vi "ICG_YY.vi"() -> ()   [LabVIEW 2020]
uses:
  <vilib>/Utility/file.llb/Read Delimited Spreadsheet (DBL).vi
  <vilib>/Analysis/NI_AALPro.lvlib
panel:
  out "size(s)":i32
  out "SV 4":dbl
  out "SV 3":dbl
  out "SV 2":dbl
  out "SV":dbl
  out "SV":dbl
  out "Tlve 5":dbl
  out "interval7 2":dbl[](graph)
  out "location 5":dbl[](array[numeric])
  out "interval 7":dbl[](array[numeric])
  out "amplitude 5":dbl[](array[numeric])
  out "Amplitudes 5":dbl[](array[numeric])
  out "2nd Derivatives 5":dbl[](array[numeric])
  out "Locations 5":dbl[](array[numeric])
  out "max  4":dbl
  out "deltaZe(t)4 2":dbl[](graph)
  out "ICG array 5":dbl[](array[numeric])
  in  "file path (dialog if empty) 5":path
  out "Tlve 4":dbl
  out "interval7":dbl[](graph)
  out "location 4":dbl[](array[numeric])
  out "interval 6":dbl[](array[numeric])
  out "amplitude 4":dbl[](array[numeric])
  out "Amplitudes 4":dbl[](array[numeric])
  out "2nd Derivatives 4":dbl[](array[numeric])
  out "Locations 4":dbl[](array[numeric])
  out "max  3":dbl
  out "deltaZe(t)4":dbl[](graph)
  out "ICG array 4":dbl[](array[numeric])
  in  "file path (dialog if empty) 4":path
  out "Tlve 3":dbl
  out "interval 5":dbl[](graph)
  out "location 3":dbl[](array[numeric])
  out "interval 4":dbl[](array[numeric])
  out "amplitude 3":dbl[](array[numeric])
  out "Amplitudes 3":dbl[](array[numeric])
  out "2nd Derivatives 3":dbl[](array[numeric])
  out "Locations 3":dbl[](array[numeric])
  out "max  2":dbl
  out "deltaZe(t) 3":dbl[](graph)
  out "ICG array 3":dbl[](array[numeric])
  in  "file path (dialog if empty) 3":path
  out "Tlve 2":dbl
  out "interval 3":dbl[](graph)
  out "location 2":dbl[](array[numeric])
  out "interval 2":dbl[](array[numeric])
  out "amplitude 2":dbl[](array[numeric])
  out "Amplitudes 2":dbl[](array[numeric])
  out "2nd Derivatives 2":dbl[](array[numeric])
  out "Locations 2":dbl[](array[numeric])
  out "max  2":dbl
  out "deltaZe(t) 2":dbl[](graph)
  out "ICG":dbl[](array[numeric])
  in  "file path (dialog if empty) 2":path
  out "Tlve":dbl
  out "interval":dbl[](graph)
  out "location":dbl[](array[numeric])
  out "interval":dbl[](array[numeric])
  out "amplitude":dbl[](array[numeric])
  out "Amplitudes":dbl[](array[numeric])
  out "2nd Derivatives":dbl[](array[numeric])
  out "Locations":dbl[](array[numeric])
  out "max":dbl
  out "deltaZe(t)":dbl[](graph)
  out "ICG":dbl[](array[numeric])
  in  "file path (dialog if empty)":path
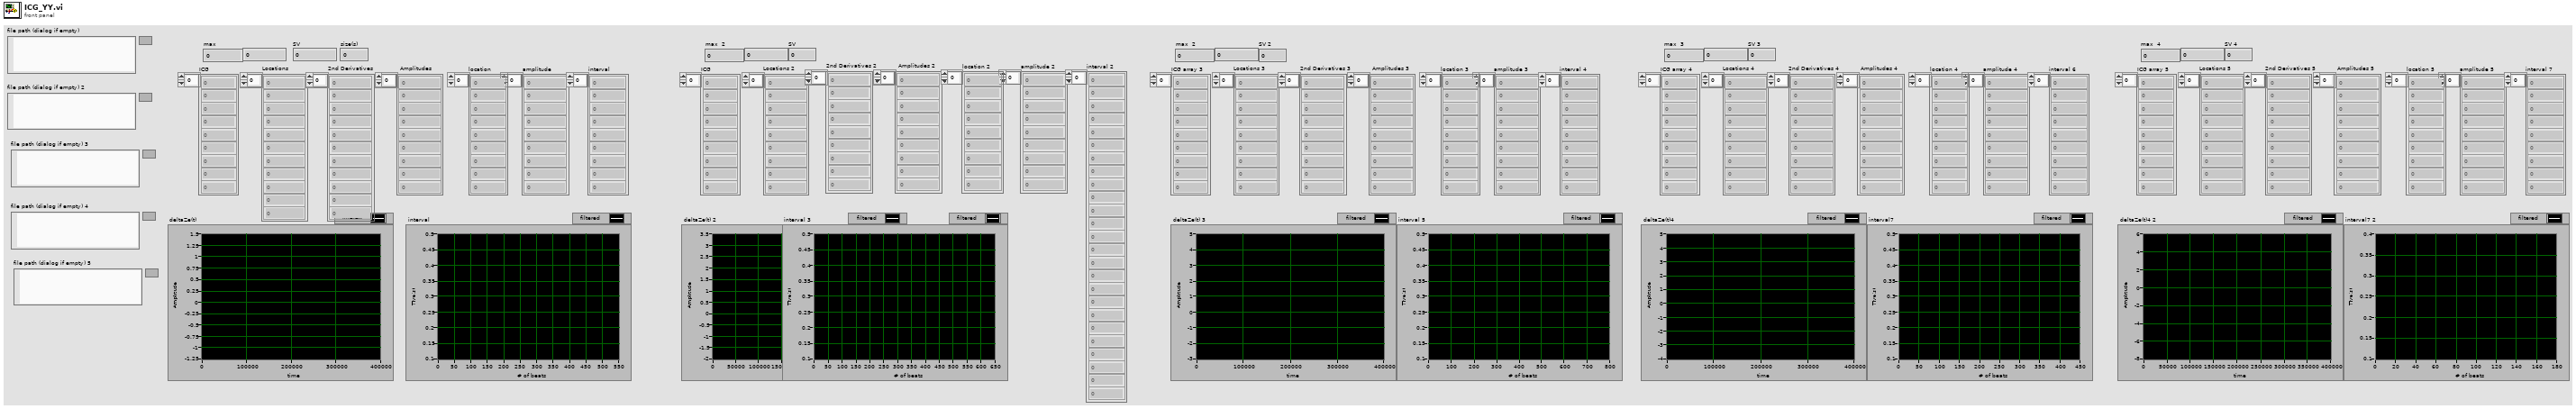
[diagram p1: front panel]
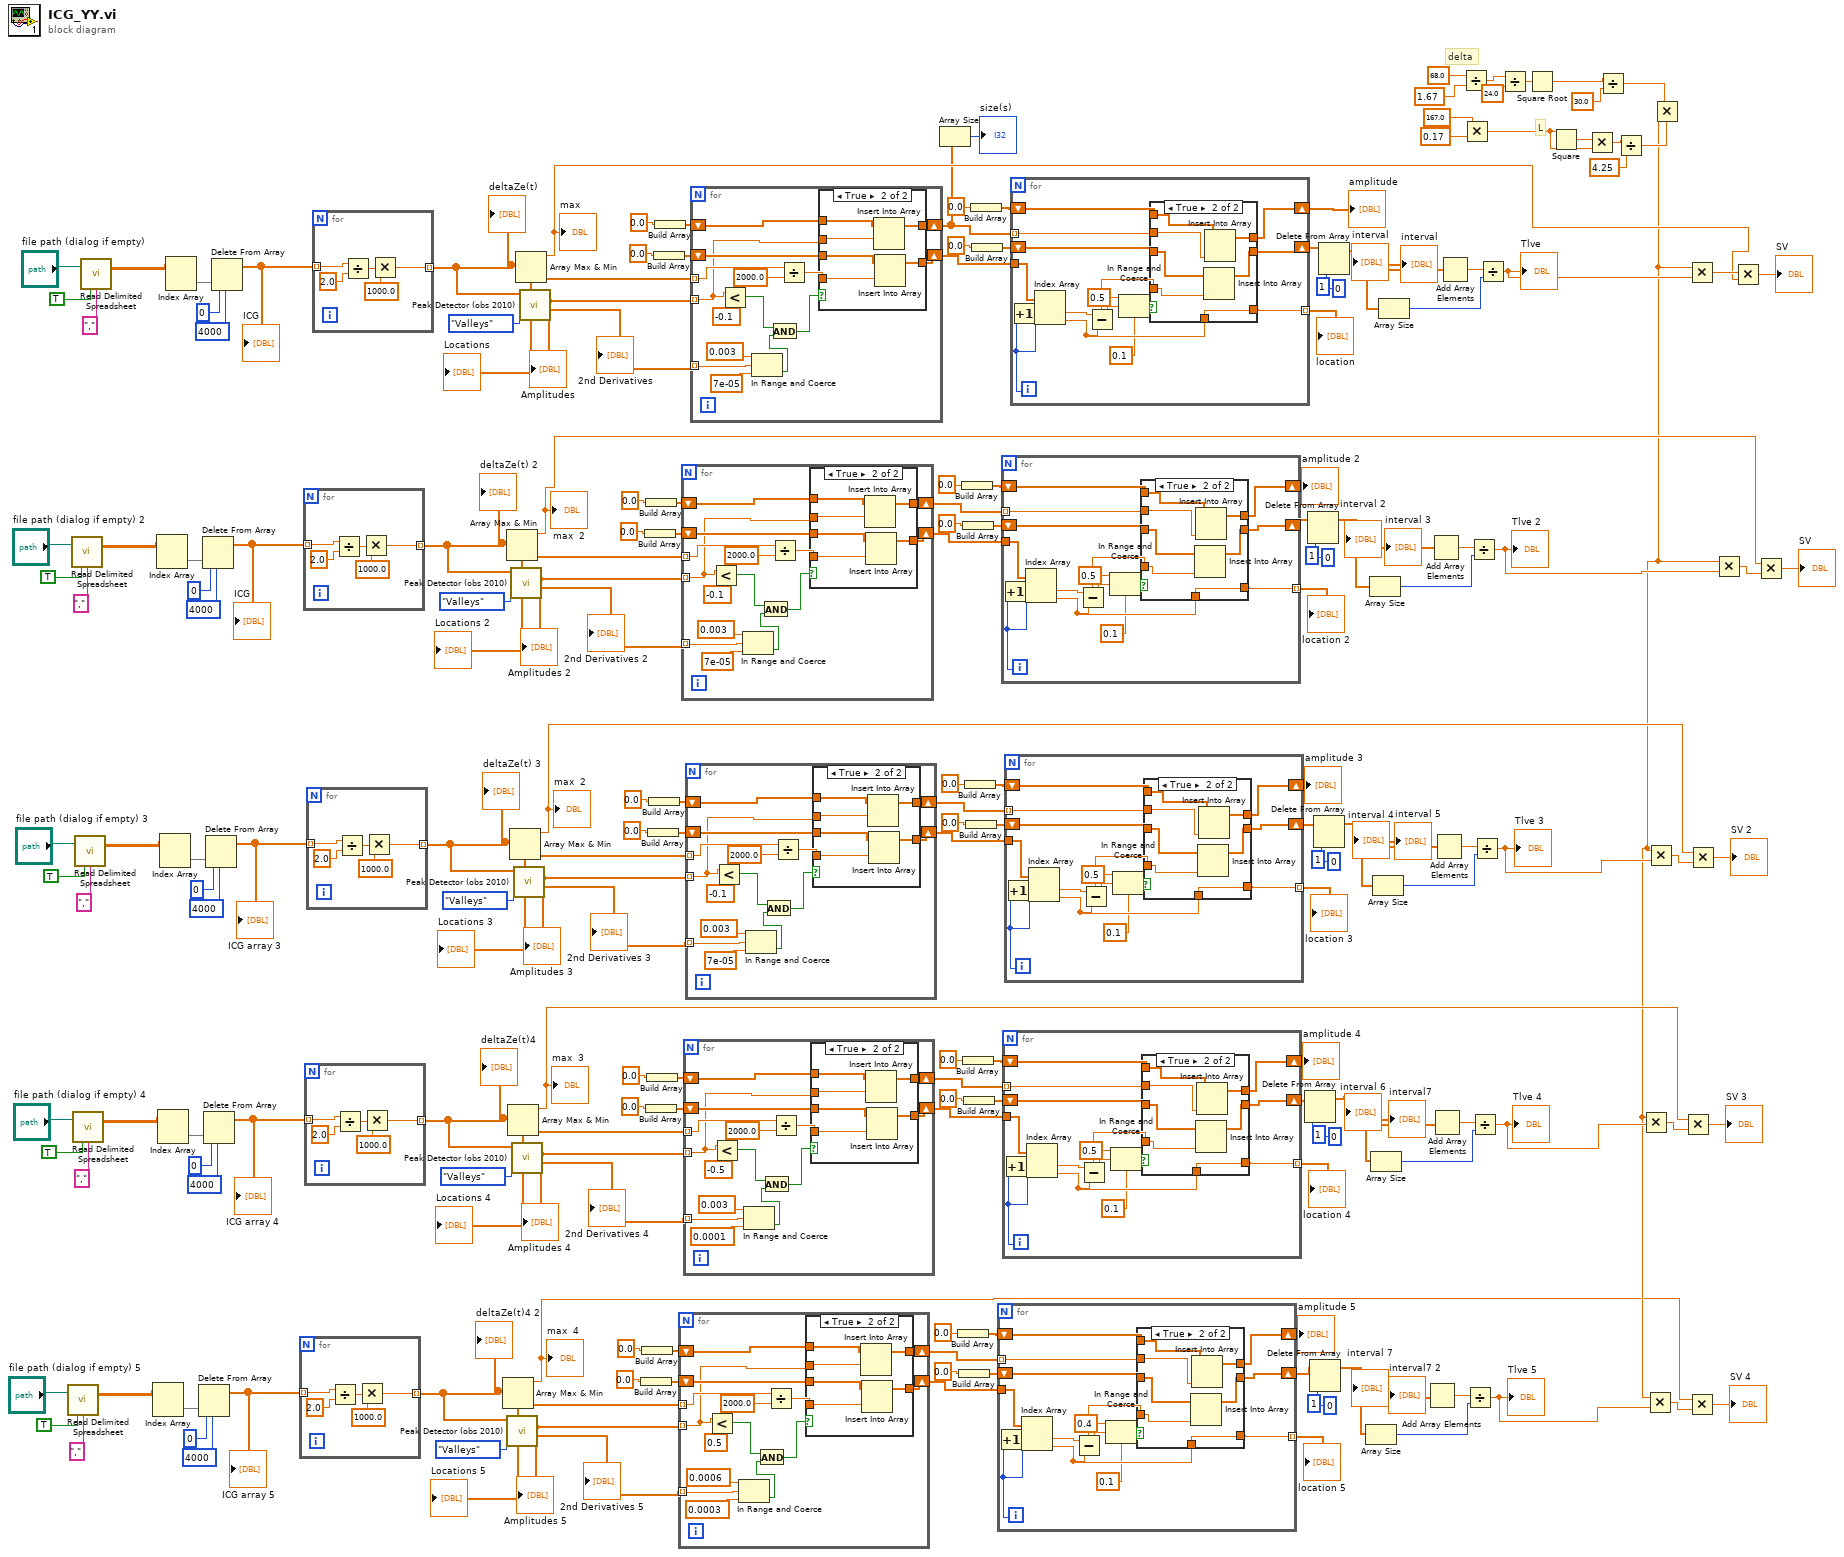
[diagram p0: block diagram]
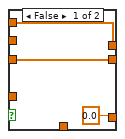
[diagram p2: hidden frame]
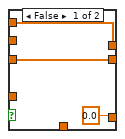
[diagram p4: hidden frame]
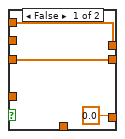
[diagram p6: hidden frame]
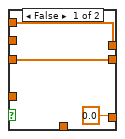
[diagram p8: hidden frame]
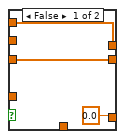
[diagram p10: hidden frame]
diagram:
  (unwired) 1 ("length")
  (unwired) 1 ("length")
  (unwired) 1 ("length")
  (unwired) 1 ("length")
  (unwired) 1 ("length")
  # "L"
  # "delta"
  n1 = call-poly <vilib>:"Read Delimited Spreadsheet.vi"("file path (dialog if empty)"="file path (dialog if empty) 5", "transpose? (F)"=TRUE, "delimiter (\\t)"="," ("delimiter (\\t)")) -> ("all rows"=w77:dbl[][])  [unwired: 7 in, 5 out]
  n2 = call-poly <vilib>:"Read Delimited Spreadsheet.vi"("file path (dialog if empty)"="file path (dialog if empty) 2", "transpose? (F)"=TRUE, "delimiter (\\t)"="," ("delimiter (\\t)")) -> ("all rows"=w158:dbl[][])  [unwired: 7 in, 5 out]
  n3 = call-poly <vilib>:"Read Delimited Spreadsheet.vi"("file path (dialog if empty)"="file path (dialog if empty) 4", "transpose? (F)"=TRUE, "delimiter (\\t)"="," ("delimiter (\\t)")) -> ("all rows"=w104:dbl[][])  [unwired: 7 in, 5 out]
  n4 = call-poly <vilib>:"Read Delimited Spreadsheet.vi"("file path (dialog if empty)"="file path (dialog if empty) 3", "transpose? (F)"=TRUE, "delimiter (\\t)"="," ("delimiter (\\t)")) -> ("all rows"=w131:dbl[][])  [unwired: 7 in, 5 out]
  n5 = call-poly <vilib>:"Read Delimited Spreadsheet.vi"("file path (dialog if empty)"="file path (dialog if empty)", "transpose? (F)"=TRUE, "delimiter (\\t)"="," ("delimiter (\\t)")) -> ("all rows"=w184:dbl[][])  [unwired: 7 in, 5 out]
  n6 = Index Array(array=w77) -> (element=w76:dbl[])  [unwired: 2 in]
  n7 = Index Array(array=w158) -> (element=w157:dbl[])  [unwired: 2 in]
  n8 = Index Array(array=w104) -> (element=w103:dbl[])  [unwired: 2 in]
  n9 = Index Array(array=w131) -> (element=w130:dbl[])  [unwired: 2 in]
  n10 = Index Array(array=w184) -> (element=w183:dbl[])  [unwired: 2 in]
  n11 = Delete From Array(array=w76, length=4000, index=0) -> (array with subset deleted=w73:dbl[])  [unwired: 1 out]
  "ICG array 5" <- w73
  n12 = Delete From Array(array=w157, length=4000, index=0) -> (array with subset deleted=w154:dbl[])  [unwired: 1 out]
  "ICG" <- w154
  n13 = Delete From Array(array=w103, length=4000, index=0) -> (array with subset deleted=w100:dbl[])  [unwired: 1 out]
  "ICG array 4" <- w100
  n14 = Delete From Array(array=w130, length=4000, index=0) -> (array with subset deleted=w127:dbl[])  [unwired: 1 out]
  "ICG array 3" <- w127
  n15 = Delete From Array(array=w183, length=4000, index=0) -> (array with subset deleted=w180:dbl[])  [unwired: 1 out]
  "ICG" <- w180
  n16 = for {
    tunnel: w73 -> [w192] mode=indexing
    tunnel: [w188] -> w69 mode=indexing
    n17 = Divide(x=w192, y=2.0) -> (x/y=w190:dbl)
    n18 = Multiply(x=w190, y=1000.0) -> (x*y=w188:dbl)
  }
  "deltaZe(t)4 2" <- w69
  n19 = for {
    tunnel: w154 -> [w197] mode=indexing
    tunnel: [w193] -> w150 mode=indexing
    n20 = Divide(x=w197, y=2.0) -> (x/y=w195:dbl)
    n21 = Multiply(x=w195, y=1000.0) -> (x*y=w193:dbl)
  }
  "deltaZe(t) 2" <- w150
  n22 = for {
    tunnel: w100 -> [w202] mode=indexing
    tunnel: [w198] -> w96 mode=indexing
    n23 = Divide(x=w202, y=2.0) -> (x/y=w200:dbl)
    n24 = Multiply(x=w200, y=1000.0) -> (x*y=w198:dbl)
  }
  "deltaZe(t)4" <- w96
  n25 = for {
    tunnel: w127 -> [w207] mode=indexing
    tunnel: [w203] -> w123 mode=indexing
    n26 = Divide(x=w207, y=2.0) -> (x/y=w205:dbl)
    n27 = Multiply(x=w205, y=1000.0) -> (x*y=w203:dbl)
  }
  "deltaZe(t) 3" <- w123
  n28 = for {
    tunnel: w180 -> [w212] mode=indexing
    tunnel: [w208] -> w176 mode=indexing
    n29 = Divide(x=w212, y=2.0) -> (x/y=w210:dbl)
    n30 = Multiply(x=w210, y=1000.0) -> (x*y=w208:dbl)
  }
  "deltaZe(t)" <- w176
  n31 = Array Max & Min(array=w69) -> (max value=w18:dbl)  [unwired: 3 out]
  "max  4" <- w18
  n32 = Array Max & Min(array=w150) -> (max value=w33:dbl)  [unwired: 3 out]
  "max  2" <- w33
  n33 = call <vilib>:"Peak Detector (obs 2010).vi"("peaks/valleys"=enum32{"Peaks", "Valleys"}."Valleys", "X"=w69) -> ("2nd Derivatives"=w67:dbl[], "Amplitudes"=w68:dbl[], "Locations"=w64:dbl[])  [unwired: 5 in, 2 out]
  "Locations 5" <- w64
  "2nd Derivatives 5" <- w67
  "Amplitudes 5" <- w68
  n34 = Array Max & Min(array=w96) -> (max value=w23:dbl)  [unwired: 3 out]
  "max  3" <- w23
  n35 = Array Max & Min(array=w123) -> (max value=w27:dbl)  [unwired: 3 out]
  "max  2" <- w27
  n36 = call <vilib>:"Peak Detector (obs 2010).vi"("peaks/valleys"=enum32{"Peaks", "Valleys"}."Valleys", "X"=w150) -> ("2nd Derivatives"=w148:dbl[], "Amplitudes"=w149:dbl[], "Locations"=w145:dbl[])  [unwired: 5 in, 2 out]
  "Locations 2" <- w145
  "2nd Derivatives 2" <- w148
  "Amplitudes 2" <- w149
  n37 = call <vilib>:"Peak Detector (obs 2010).vi"("peaks/valleys"=enum32{"Peaks", "Valleys"}."Valleys", "X"=w96) -> ("2nd Derivatives"=w94:dbl[], "Amplitudes"=w95:dbl[], "Locations"=w91:dbl[])  [unwired: 5 in, 2 out]
  "Locations 4" <- w91
  "2nd Derivatives 4" <- w94
  "Amplitudes 4" <- w95
  n38 = call <vilib>:"Peak Detector (obs 2010).vi"("peaks/valleys"=enum32{"Peaks", "Valleys"}."Valleys", "X"=w123) -> ("2nd Derivatives"=w121:dbl[], "Amplitudes"=w122:dbl[], "Locations"=w118:dbl[])  [unwired: 5 in, 2 out]
  "Locations 3" <- w118
  "2nd Derivatives 3" <- w121
  "Amplitudes 3" <- w122
  n39 = Array Max & Min(array=w176) -> (max value=w35:dbl)  [unwired: 3 out]
  "max" <- w35
  n40 = call <vilib>:"Peak Detector (obs 2010).vi"("peaks/valleys"=enum32{"Peaks", "Valleys"}."Valleys", "X"=w176) -> ("2nd Derivatives"=w174:dbl[], "Amplitudes"=w175:dbl[], "Locations"=w171:dbl[])  [unwired: 5 in, 2 out]
  "Locations" <- w171
  "2nd Derivatives" <- w174
  "Amplitudes" <- w175
  n41 = Build Array(0.0 ("array")) -> (w65:dbl[])
  n42 = Build Array(0.0 ("array")) -> (w70:dbl[])
  n43 = Build Array(0.0 ("array")) -> (w146:dbl[])
  n44 = Build Array(0.0 ("array")) -> (w151:dbl[])
  n45 = Build Array(0.0 ("array")) -> (w92:dbl[])
  n46 = Build Array(0.0 ("array")) -> (w97:dbl[])
  n47 = Build Array(0.0 ("array")) -> (w119:dbl[])
  n48 = Build Array(0.0 ("array")) -> (w124:dbl[])
  n49 = Build Array(0.0 ("array")) -> (w172:dbl[])
  n50 = Build Array(0.0 ("array")) -> (w177:dbl[])
  n51 = for {
    tunnel: w68 -> [w213] mode=indexing
    shift-right: [w225] -> w63
    shift-left: w70 -> [w226]
    tunnel: w67 -> [w220] mode=indexing
    shift-right: [w218] -> w62
    shift-left: w65 -> [w219]
    tunnel: w64 -> [w216] mode=indexing
    n52 = Less?(x=w213, y=0.5) -> (x < y?=w222:bool)
    n53 = In Range and Coerce(upper limit=0.0006, x=w220, lower limit=0.0003) -> (In Range?=w217:bool)  [unwired: 1 out]
    n54 = And(x=w222, y=w217) -> (x .and. y?=w221:bool)
    n55 = Divide(x=w216, y=2000.0) -> (x/y=w214:dbl)
    n56 = case shown="True" w221 {
      tunnel: w226 -> [w229 w235]
      tunnel: [w229 w234] -> w225
      tunnel: w213 -> [_ w233]
      tunnel: w219 -> [w228 w232]
      tunnel: [w228 w231] -> w218
      tunnel: w214 -> [_ w230]
      frame False {
      }
      frame True {
        n57 = Insert Into Array(array=w235, new element=w233) -> (w234:dbl[])  [unwired: 1 in]
        n58 = Insert Into Array(array=w232, new element=w230) -> (w231:dbl[])  [unwired: 1 in]
      }
    }
  }
  n59 = for {
    tunnel: w149 -> [w236] mode=indexing
    shift-right: [w248] -> w144
    shift-left: w151 -> [w249]
    tunnel: w148 -> [w243] mode=indexing
    shift-right: [w241] -> w143
    shift-left: w146 -> [w242]
    tunnel: w145 -> [w239] mode=indexing
    n60 = Less?(x=w236, y=-0.1) -> (x < y?=w245:bool)
    n61 = In Range and Coerce(upper limit=0.003, x=w243, lower limit=7e-05) -> (In Range?=w240:bool)  [unwired: 1 out]
    n62 = And(x=w245, y=w240) -> (x .and. y?=w244:bool)
    n63 = Divide(x=w239, y=2000.0) -> (x/y=w237:dbl)
    n64 = case shown="True" w244 {
      tunnel: w249 -> [w252 w258]
      tunnel: [w252 w257] -> w248
      tunnel: w236 -> [_ w256]
      tunnel: w242 -> [w251 w255]
      tunnel: [w251 w254] -> w241
      tunnel: w237 -> [_ w253]
      frame False {
      }
      frame True {
        n65 = Insert Into Array(array=w258, new element=w256) -> (w257:dbl[])  [unwired: 1 in]
        n66 = Insert Into Array(array=w255, new element=w253) -> (w254:dbl[])  [unwired: 1 in]
      }
    }
  }
  n67 = for {
    tunnel: w95 -> [w259] mode=indexing
    shift-right: [w271] -> w90
    shift-left: w97 -> [w272]
    tunnel: w94 -> [w266] mode=indexing
    shift-right: [w264] -> w89
    shift-left: w92 -> [w265]
    tunnel: w91 -> [w262] mode=indexing
    n68 = Less?(x=w259, y=-0.5) -> (x < y?=w268:bool)
    n69 = In Range and Coerce(upper limit=0.003, x=w266, lower limit=0.0001) -> (In Range?=w263:bool)  [unwired: 1 out]
    n70 = And(x=w268, y=w263) -> (x .and. y?=w267:bool)
    n71 = Divide(x=w262, y=2000.0) -> (x/y=w260:dbl)
    n72 = case shown="True" w267 {
      tunnel: w272 -> [w275 w281]
      tunnel: [w275 w280] -> w271
      tunnel: w259 -> [_ w279]
      tunnel: w265 -> [w274 w278]
      tunnel: [w274 w277] -> w264
      tunnel: w260 -> [_ w276]
      frame False {
      }
      frame True {
        n73 = Insert Into Array(array=w281, new element=w279) -> (w280:dbl[])  [unwired: 1 in]
        n74 = Insert Into Array(array=w278, new element=w276) -> (w277:dbl[])  [unwired: 1 in]
      }
    }
  }
  n75 = for {
    tunnel: w122 -> [w282] mode=indexing
    shift-right: [w294] -> w117
    shift-left: w124 -> [w295]
    tunnel: w121 -> [w289] mode=indexing
    shift-right: [w287] -> w116
    shift-left: w119 -> [w288]
    tunnel: w118 -> [w285] mode=indexing
    n76 = Less?(x=w282, y=-0.1) -> (x < y?=w291:bool)
    n77 = In Range and Coerce(upper limit=0.003, x=w289, lower limit=7e-05) -> (In Range?=w286:bool)  [unwired: 1 out]
    n78 = And(x=w291, y=w286) -> (x .and. y?=w290:bool)
    n79 = Divide(x=w285, y=2000.0) -> (x/y=w283:dbl)
    n80 = case shown="True" w290 {
      tunnel: w295 -> [w298 w304]
      tunnel: [w298 w303] -> w294
      tunnel: w282 -> [_ w302]
      tunnel: w288 -> [w297 w301]
      tunnel: [w297 w300] -> w287
      tunnel: w283 -> [_ w299]
      frame False {
      }
      frame True {
        n81 = Insert Into Array(array=w304, new element=w302) -> (w303:dbl[])  [unwired: 1 in]
        n82 = Insert Into Array(array=w301, new element=w299) -> (w300:dbl[])  [unwired: 1 in]
      }
    }
  }
  n83 = for {
    tunnel: w175 -> [w305] mode=indexing
    shift-right: [w317] -> w17
    shift-left: w177 -> [w318]
    tunnel: w174 -> [w312] mode=indexing
    shift-right: [w310] -> w170
    shift-left: w172 -> [w311]
    tunnel: w171 -> [w308] mode=indexing
    n84 = Less?(x=w305, y=-0.1) -> (x < y?=w314:bool)
    n85 = In Range and Coerce(upper limit=0.003, x=w312, lower limit=7e-05) -> (In Range?=w309:bool)  [unwired: 1 out]
    n86 = And(x=w314, y=w309) -> (x .and. y?=w313:bool)
    n87 = Divide(x=w308, y=2000.0) -> (x/y=w306:dbl)
    n88 = case shown="True" w313 {
      tunnel: w318 -> [w321 w327]
      tunnel: [w321 w326] -> w317
      tunnel: w305 -> [_ w325]
      tunnel: w311 -> [w320 w324]
      tunnel: [w320 w323] -> w310
      tunnel: w306 -> [_ w322]
      frame False {
      }
      frame True {
        n89 = Insert Into Array(array=w327, new element=w325) -> (w326:dbl[])  [unwired: 1 in]
        n90 = Insert Into Array(array=w324, new element=w322) -> (w323:dbl[])  [unwired: 1 in]
      }
    }
  }
  n91 = Array Size(array=w17) -> (size(s)=→"size(s)":i32)
  n92 = Build Array(0.0 ("array")) -> (w59:dbl[])
  n93 = Build Array(0.0 ("array")) -> (w60:dbl[])
  n94 = Build Array(0.0 ("array")) -> (w140:dbl[])
  n95 = Build Array(0.0 ("array")) -> (w141:dbl[])
  n96 = Build Array(0.0 ("array")) -> (w86:dbl[])
  n97 = Build Array(0.0 ("array")) -> (w87:dbl[])
  n98 = Build Array(0.0 ("array")) -> (w113:dbl[])
  n99 = Build Array(0.0 ("array")) -> (w114:dbl[])
  n100 = Build Array(0.0 ("array")) -> (w167:dbl[])
  n101 = Build Array(0.0 ("array")) -> (w168:dbl[])
  n102 = for {
    tunnel: w62 -> [w340]
    shift-right: [w336] -> w2
    shift-left: w60 -> [w337]
    tunnel: w63 -> [w332] mode=indexing
    shift-right: [w342] -> w57
    shift-left: w59 -> [w335]
    tunnel: [w333] -> w56 mode=indexing
    i -> [w339]
    n103 = Increment(x=w339) -> (x+1=w341:i32)
    n104 = Index Array(array=w340, index #1=w341, index #2=w339) -> (element #1=w338:dbl, element #2=w334:dbl)
    n105 = Subtract(x=w338, y=w334) -> (x-y=w328:dbl)
    n106 = In Range and Coerce(upper limit=0.4, x=w328, lower limit=0.1 ("y")) -> (In Range?=w331:bool)  [unwired: 1 out]
    n107 = case shown="True" w331 {
      tunnel: w332 -> [_ w348]
      tunnel: [w344 w352] -> w342
      tunnel: w337 -> [w345 w351]
      tunnel: [w345 w350] -> w336
      tunnel: w335 -> [w344 w349]
      tunnel: w328 -> [_ w347]
      tunnel: w334 -> [_ w346]
      tunnel: [0.0 ("array") w346] -> w333
      frame False {
      }
      frame True {
        n108 = Insert Into Array(array=w351, new element=w347) -> (w350:dbl[])  [unwired: 1 in]
        n109 = Insert Into Array(array=w349, new element=w348) -> (w352:dbl[])  [unwired: 1 in]
      }
    }
  }
  "amplitude 5" <- w57
  "location 5" <- w56
  n110 = for {
    tunnel: w143 -> [w365]
    shift-right: [w361] -> w11
    shift-left: w141 -> [w362]
    tunnel: w144 -> [w357] mode=indexing
    shift-right: [w367] -> w138
    shift-left: w140 -> [w360]
    tunnel: [w358] -> w137 mode=indexing
    i -> [w364]
    n111 = Increment(x=w364) -> (x+1=w366:i32)
    n112 = Index Array(array=w365, index #1=w366, index #2=w364) -> (element #1=w363:dbl, element #2=w359:dbl)
    n113 = Subtract(x=w363, y=w359) -> (x-y=w353:dbl)
    n114 = In Range and Coerce(upper limit=0.5, x=w353, lower limit=0.1 ("y")) -> (In Range?=w356:bool)  [unwired: 1 out]
    n115 = case shown="True" w356 {
      tunnel: w357 -> [_ w373]
      tunnel: [w369 w377] -> w367
      tunnel: w362 -> [w370 w376]
      tunnel: [w370 w375] -> w361
      tunnel: w360 -> [w369 w374]
      tunnel: w353 -> [_ w372]
      tunnel: w359 -> [_ w371]
      tunnel: [0.0 ("array") w371] -> w358
      frame False {
      }
      frame True {
        n116 = Insert Into Array(array=w376, new element=w372) -> (w375:dbl[])  [unwired: 1 in]
        n117 = Insert Into Array(array=w374, new element=w373) -> (w377:dbl[])  [unwired: 1 in]
      }
    }
  }
  "amplitude 2" <- w138
  "location 2" <- w137
  n118 = for {
    tunnel: w89 -> [w390]
    shift-right: [w386] -> w5
    shift-left: w87 -> [w387]
    tunnel: w90 -> [w382] mode=indexing
    shift-right: [w392] -> w84
    shift-left: w86 -> [w385]
    tunnel: [w383] -> w83 mode=indexing
    i -> [w389]
    n119 = Increment(x=w389) -> (x+1=w391:i32)
    n120 = Index Array(array=w390, index #1=w391, index #2=w389) -> (element #1=w388:dbl, element #2=w384:dbl)
    n121 = Subtract(x=w388, y=w384) -> (x-y=w378:dbl)
    n122 = In Range and Coerce(upper limit=0.5, x=w378, lower limit=0.1 ("y")) -> (In Range?=w381:bool)  [unwired: 1 out]
    n123 = case shown="True" w381 {
      tunnel: w382 -> [_ w398]
      tunnel: [w394 w402] -> w392
      tunnel: w387 -> [w395 w401]
      tunnel: [w395 w400] -> w386
      tunnel: w385 -> [w394 w399]
      tunnel: w378 -> [_ w397]
      tunnel: w384 -> [_ w396]
      tunnel: [0.0 ("array") w396] -> w383
      frame False {
      }
      frame True {
        n124 = Insert Into Array(array=w401, new element=w397) -> (w400:dbl[])  [unwired: 1 in]
        n125 = Insert Into Array(array=w399, new element=w398) -> (w402:dbl[])  [unwired: 1 in]
      }
    }
  }
  "amplitude 4" <- w84
  "location 4" <- w83
  n126 = for {
    tunnel: w116 -> [w415]
    shift-right: [w411] -> w8
    shift-left: w114 -> [w412]
    tunnel: w117 -> [w407] mode=indexing
    shift-right: [w417] -> w111
    shift-left: w113 -> [w410]
    tunnel: [w408] -> w110 mode=indexing
    i -> [w414]
    n127 = Increment(x=w414) -> (x+1=w416:i32)
    n128 = Index Array(array=w415, index #1=w416, index #2=w414) -> (element #1=w413:dbl, element #2=w409:dbl)
    n129 = Subtract(x=w413, y=w409) -> (x-y=w403:dbl)
    n130 = In Range and Coerce(upper limit=0.5, x=w403, lower limit=0.1 ("y")) -> (In Range?=w406:bool)  [unwired: 1 out]
    n131 = case shown="True" w406 {
      tunnel: w407 -> [_ w423]
      tunnel: [w419 w427] -> w417
      tunnel: w412 -> [w420 w426]
      tunnel: [w420 w425] -> w411
      tunnel: w410 -> [w419 w424]
      tunnel: w403 -> [_ w422]
      tunnel: w409 -> [_ w421]
      tunnel: [0.0 ("array") w421] -> w408
      frame False {
      }
      frame True {
        n132 = Insert Into Array(array=w426, new element=w422) -> (w425:dbl[])  [unwired: 1 in]
        n133 = Insert Into Array(array=w424, new element=w423) -> (w427:dbl[])  [unwired: 1 in]
      }
    }
  }
  "amplitude 3" <- w111
  "location 3" <- w110
  n134 = for {
    tunnel: w170 -> [w440]
    shift-right: [w428] -> w15
    shift-left: w168 -> [w437]
    tunnel: w17 -> [w433] mode=indexing
    shift-right: [w442] -> w165
    shift-left: w167 -> [w436]
    tunnel: [w434] -> w164 mode=indexing
    i -> [w439]
    n135 = Increment(x=w439) -> (x+1=w441:i32)
    n136 = Index Array(array=w440, index #1=w441, index #2=w439) -> (element #1=w438:dbl, element #2=w435:dbl)
    n137 = Subtract(x=w438, y=w435) -> (x-y=w429:dbl)
    n138 = In Range and Coerce(upper limit=0.5, x=w429, lower limit=0.1 ("y")) -> (In Range?=w432:bool)  [unwired: 1 out]
    n139 = case shown="True" w432 {
      tunnel: w433 -> [_ w448]
      tunnel: [w444 w452] -> w442
      tunnel: w437 -> [w445 w451]
      tunnel: [w445 w450] -> w428
      tunnel: w436 -> [w444 w449]
      tunnel: w429 -> [_ w447]
      tunnel: w435 -> [_ w446]
      tunnel: [0.0 ("array") w446] -> w434
      frame False {
      }
      frame True {
        n140 = Insert Into Array(array=w451, new element=w447) -> (w450:dbl[])  [unwired: 1 in]
        n141 = Insert Into Array(array=w449, new element=w448) -> (w452:dbl[])  [unwired: 1 in]
      }
    }
  }
  "amplitude" <- w165
  "location" <- w164
  n142 = Delete From Array(array=w5, index=0) -> (array with subset deleted=w4:dbl[])  [unwired: 1 in, 1 out]
  "interval 6" <- w4
  "interval7" <- w4
  n143 = Delete From Array(array=w11, index=0) -> (array with subset deleted=w10:dbl[])  [unwired: 1 in, 1 out]
  "interval 2" <- w10
  "interval 3" <- w10
  n144 = Delete From Array(array=w2, index=0) -> (array with subset deleted=w1:dbl[])  [unwired: 1 in, 1 out]
  "interval 7" <- w1
  "interval7 2" <- w1
  n145 = Delete From Array(array=w8, index=0) -> (array with subset deleted=w7:dbl[])  [unwired: 1 in, 1 out]
  "interval 4" <- w7
  "interval 5" <- w7
  n146 = Delete From Array(array=w15, index=0) -> (array with subset deleted=w13:dbl[])  [unwired: 1 in, 1 out]
  "interval" <- w13
  "interval" <- w13
  n147 = Array Size(array=w1) -> (size(s)=w54:i32)
  n148 = Array Size(array=w10) -> (size(s)=w135:i32)
  n149 = Array Size(array=w4) -> (size(s)=w81:i32)
  n150 = Array Size(array=w7) -> (size(s)=w108:i32)
  n151 = Array Size(array=w13) -> (size(s)=w162:i32)
  n152 = Add Array Elements(numeric array=w1) -> (sum=w55:dbl)
  n153 = Add Array Elements(numeric array=w10) -> (sum=w136:dbl)
  n154 = Add Array Elements(numeric array=w4) -> (sum=w82:dbl)
  n155 = Add Array Elements(numeric array=w7) -> (sum=w109:dbl)
  n156 = Add Array Elements(numeric array=w13) -> (sum=w163:dbl)
  n157 = Divide(x=68.0, y=1.67) -> (x/y=w41:dbl)
  n158 = Multiply(x=167.0, y=0.17) -> (x*y=w48:dbl)
  n159 = Divide(x=w55, y=w54) -> (x/y=w20:dbl)
  "Tlve 5" <- w20
  n160 = Divide(x=w136, y=w135) -> (x/y=w34:dbl)
  "Tlve 2" <- w34
  n161 = Divide(x=w82, y=w81) -> (x/y=w24:dbl)
  "Tlve 4" <- w24
  n162 = Divide(x=w109, y=w108) -> (x/y=w28:dbl)
  "Tlve 3" <- w28
  n163 = Divide(x=w163, y=w162) -> (x/y=w44:dbl)
  "Tlve" <- w44
  n164 = Divide(x=w41, y=24.0) -> (x/y=w39:dbl)
  n165 = Square Root(x=w39) -> (sqrt(x)=w37:dbl)
  n166 = Square(x=w48) -> (x^2=w49:dbl)
  n167 = Multiply(x=w49, y=w48) -> (x*y=w47:dbl)
  n168 = Divide(x=w37, y=30.0) -> (x/y=w46:dbl)
  n169 = Divide(x=w47, y=4.25) -> (x/y=w45:dbl)
  n170 = Multiply(x=w46, y=w45) -> (x*y=w19:dbl)
  n171 = Multiply(x=w19, y=w24) -> (x*y=w26:dbl)
  n172 = Multiply(x=w19, y=w20) -> (x*y=w22:dbl)
  n173 = Multiply(x=w19, y=w28) -> (x*y=w30:dbl)
  n174 = Multiply(x=w23, y=w26) -> (x*y=→"SV 3":dbl)
  n175 = Multiply(x=w19, y=w44) -> (x*y=w43:dbl)
  n176 = Multiply(x=w18, y=w22) -> (x*y=→"SV 4":dbl)
  n177 = Multiply(x=w27, y=w30) -> (x*y=→"SV 2":dbl)
  n178 = Multiply(x=w19, y=w34) -> (x*y=w32:dbl)
  n179 = Multiply(x=w43, y=w35) -> (x*y=→"SV":dbl)
  n180 = Multiply(x=w33, y=w32) -> (x*y=→"SV":dbl)
